vi "DOOR_ASSIGN.vi"(8 "error In":errorcluster) -> (0 "error out":errorcluster)   [LabVIEW 2017]
uses:
  Controls/Ass. Loop Control.ctl
  <vilib>/Utility/error.llb/DialogType.ctl
  <vilib>/Utility/file.llb/Read Delimited Spreadsheet (string).vi
  <vilib>/Utility/file.llb/Write Delimited Spreadsheet (string).vi
  <vilib>/Utility/config.llb/NI_LVConfig.lvlib
panel:
  in  "REMOVE PART":bool
  in  "ADD PART":bool
  in  "LIST OF PARTS":string(combo)
  in  "DOORS":string(combo)
  in  "DOORS":enum32{"ADD PARTS", "Page 1", "Page 2"}(tab)
  in  "ADDED PART LIST":string(combo)
  in  "REMOVE PART FROM LIST":bool
  in  "ADD PART IN LIST":bool
  in  "NEW PARTS BARCODE":string
  out "DOOR 1":string[](array[string])
  out "DOOR 2":string[](array[string])
  out "DOOR 3":string[](array[string])
  out "DOOR 4":string[](array[string])
  out "DOOR 5":string[](array[string])
  out "DOOR 16":string[](array[string])
  out "DOOR 11":string[](array[string])
  out "DOOR 12":string[](array[string])
  out "DOOR 13":string[](array[string])
  out "DOOR 14":string[](array[string])
  out "DOOR 15":string[](array[string])
  out "USER:-":string
  in  "Stop":bool
  out "DATE/TIME":string
  out "Screen Name":string
  # "Nm"
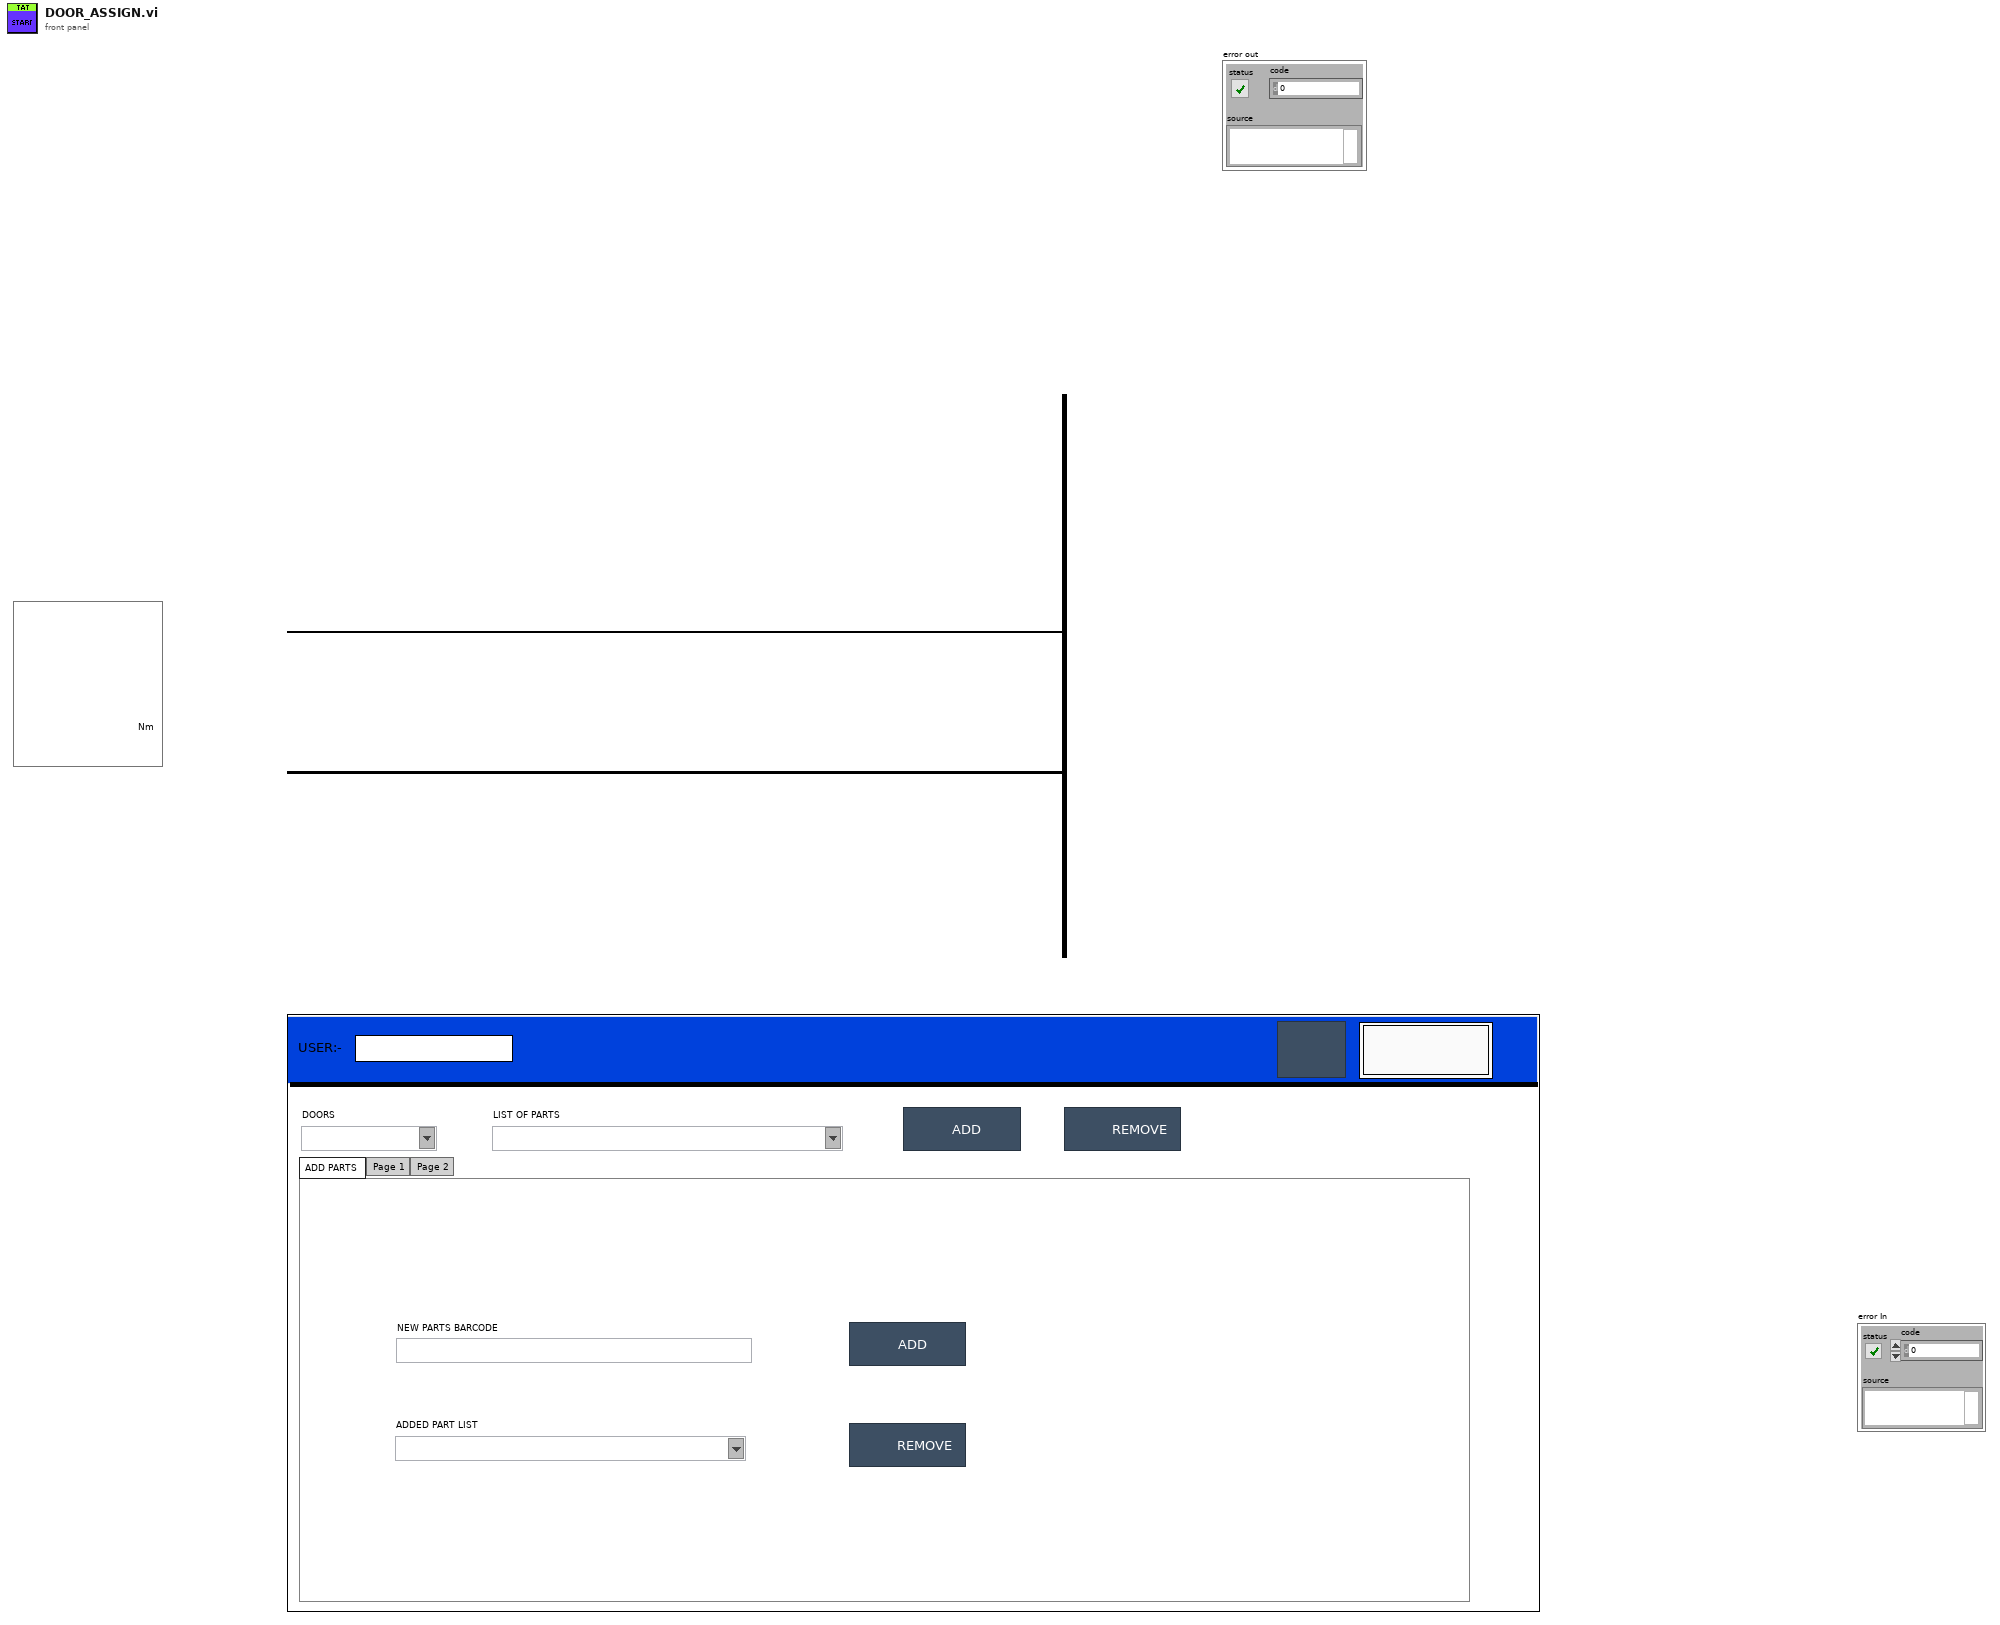
[diagram p1: front panel]
types:
  T1 = cluster{"DOOR ASSIGN":path, "PART LIST":path, "DOOR PART ASSIGN":cluster{"DOOR 1":cluster{"DOOR 1":string[]}, "DOOR 2":cluster{"DOOR 2":string[]}, "DOOR 3":cluster{"DOOR 3":string[]}, "DOOR 4":cluster{"DOOR 4":string[]}, "DOOR 5":cluster{"DOOR 5":string[]}, "DOOR 11":cluster{"DOOR 11":string[]}, "DOOR 12":cluster{"DOOR 12":string[]}, "DOOR 13":cluster{"DOOR 13":string[]}, "DOOR 14":cluster{"DOOR 14":string[]}, "DOOR 15":cluster{"DOOR 15":string[]}, "DOOR 16":cluster{"DOOR 16":string[]}}}
  T2 = typedef "Ass. Loop Control.ctl" = enum16{"Package_Qty_Count", "GENERATE_QR_PRNT", "Cluster_update", "Waiting_for_scan", "barcode CHECK", "Int", "SaveReport ", "Barcode Print", "Start Cycle", "Wait", "Cycle End", "Stop"}
  T3 = typedef "DialogType.ctl" = u16
  T4 = enum32{"invalid app kind", "Development System", "Run Time System", "Student Edition", "Embedded LabVIEW", "Evaluation", "Custom"}
  T5 = cluster{"DOOR 1":string[], "DOOR 2":string[], "DOOR 3":string[], "DOOR 4":string[], "DOOR 5":string[], "DOOR 11":string[], "DOOR 12":string[], "DOOR 13":string[], "DOOR 14":string[], "DOOR 15":string[], "DOOR 16":string[]}
  T6 = typedef "LVComboBoxStrsAndValuesArrayTypeDef.ctl" = cluster{"String":string, "Value":string}[]
  T7 = typedef "NI_LVConfig.lvlib/Config Data RefNum.ctl" = refnum<k1>
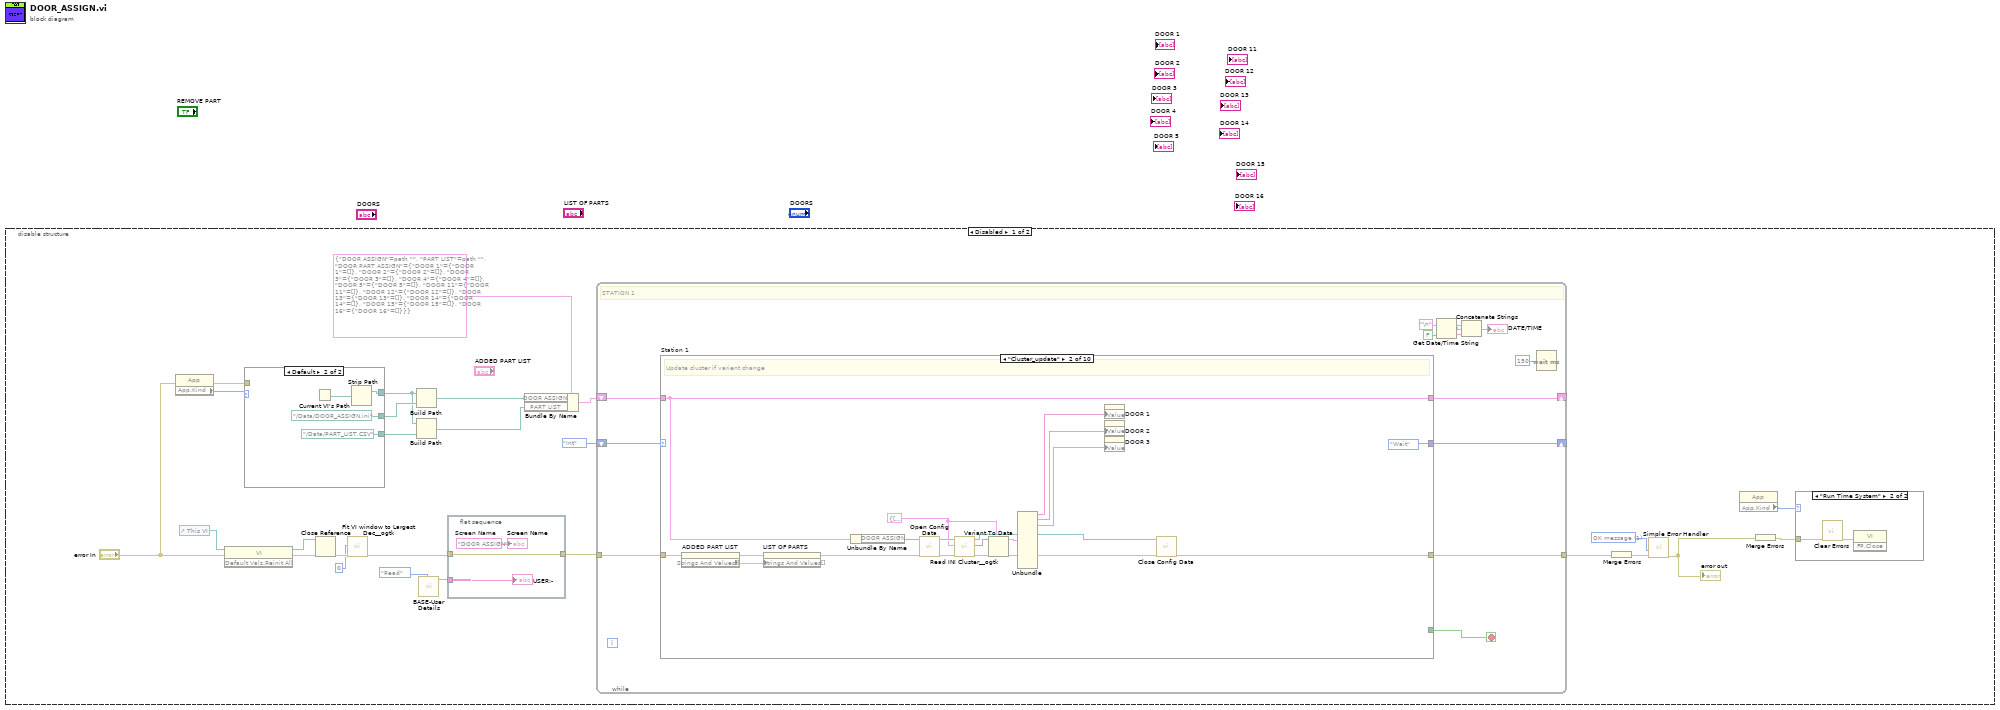
[diagram p0: block diagram]
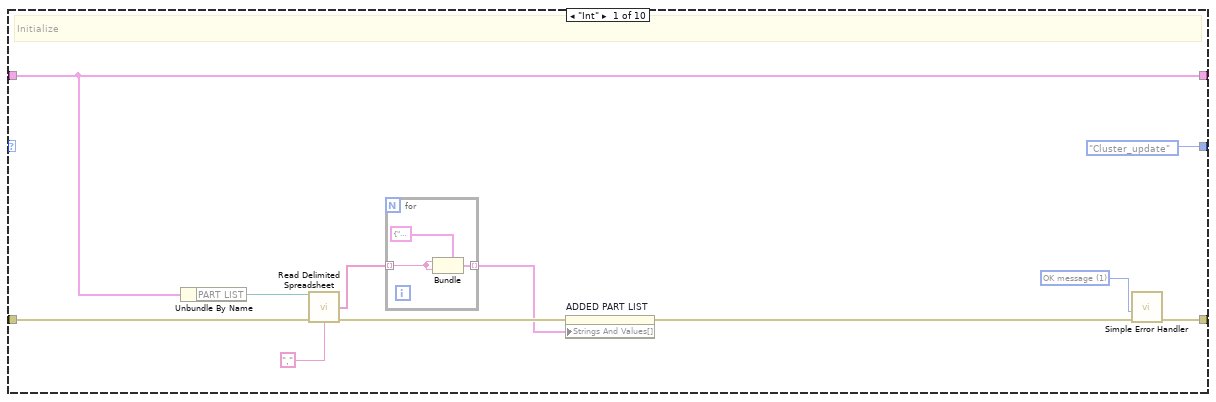
[diagram p3: hidden frame]
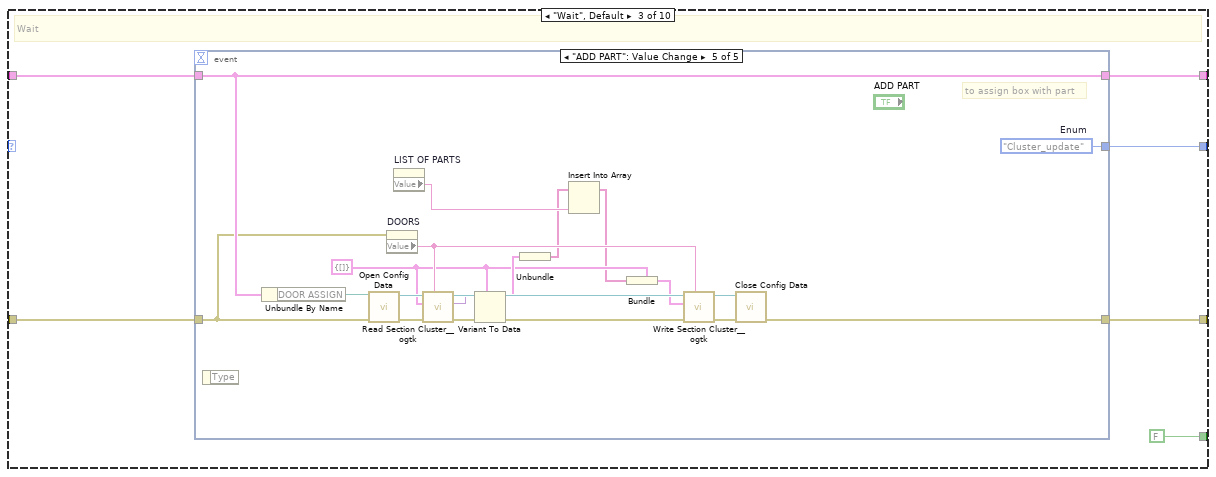
[diagram p4: hidden frame]
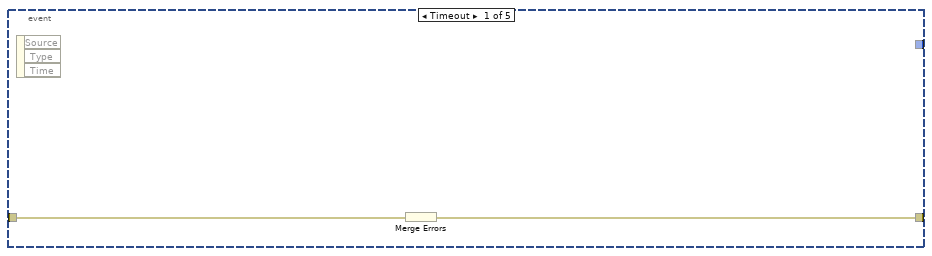
[diagram p5: hidden frame]
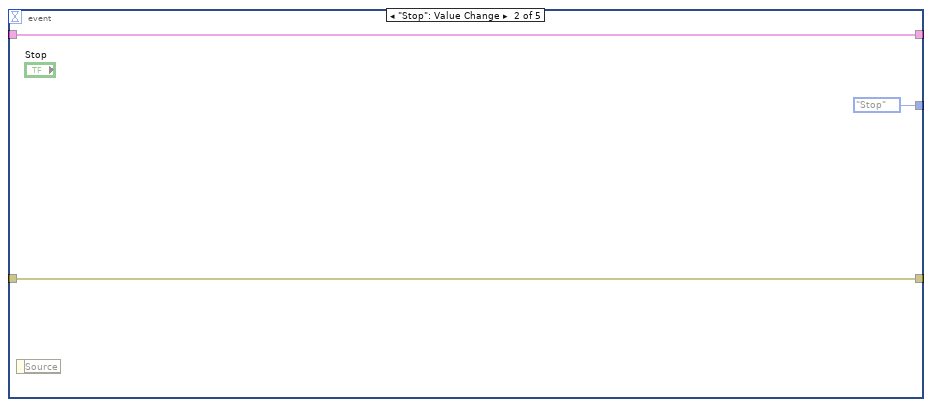
[diagram p6: hidden frame]
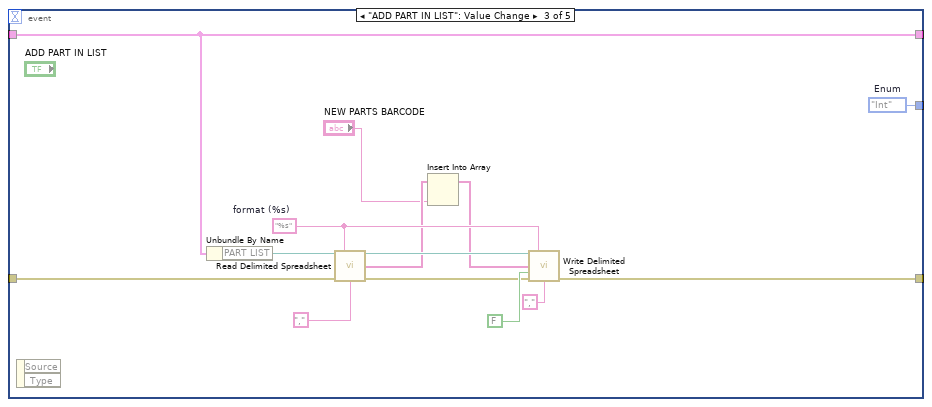
[diagram p7: hidden frame]
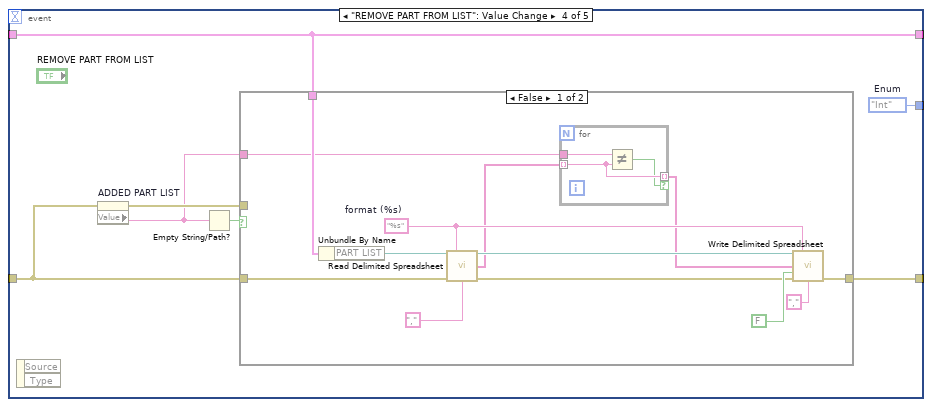
[diagram p8: hidden frame]
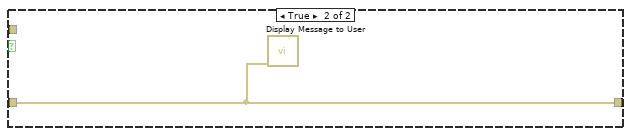
[diagram p9: hidden frame]
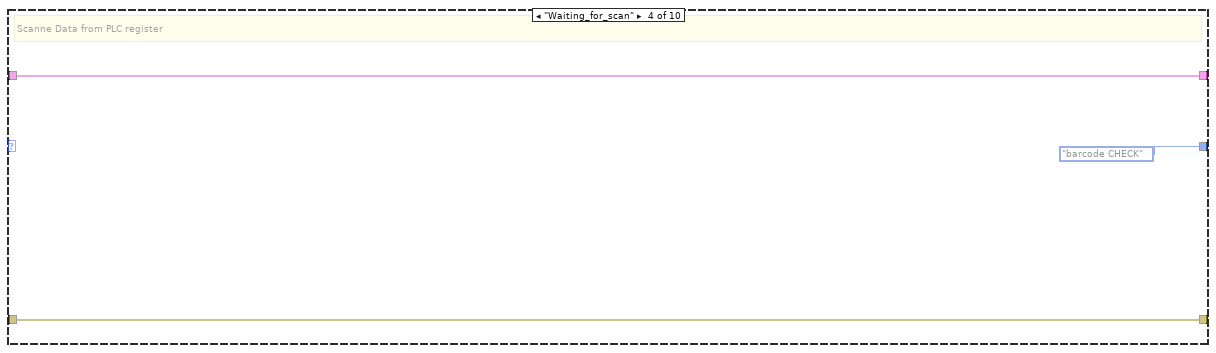
[diagram p10: hidden frame]
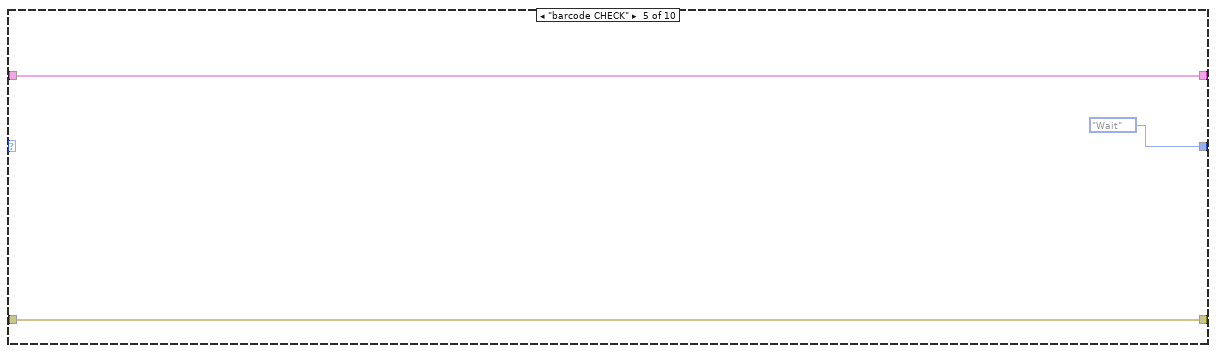
[diagram p11: hidden frame]
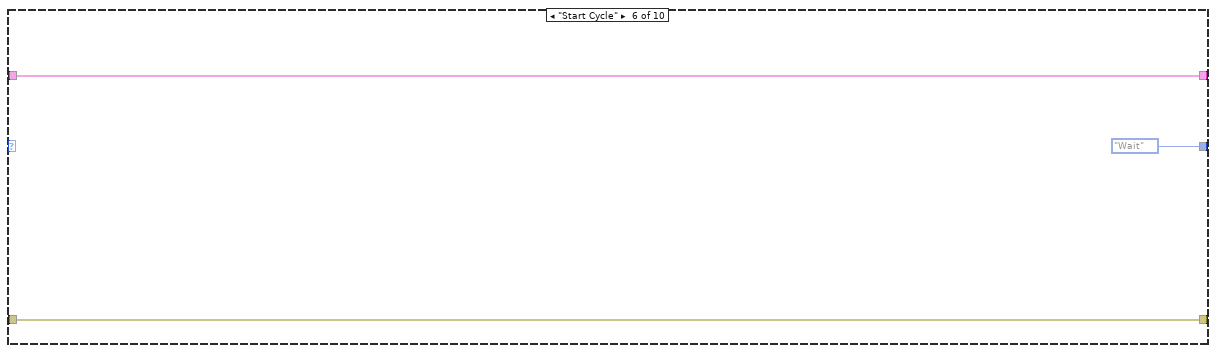
[diagram p12: hidden frame]
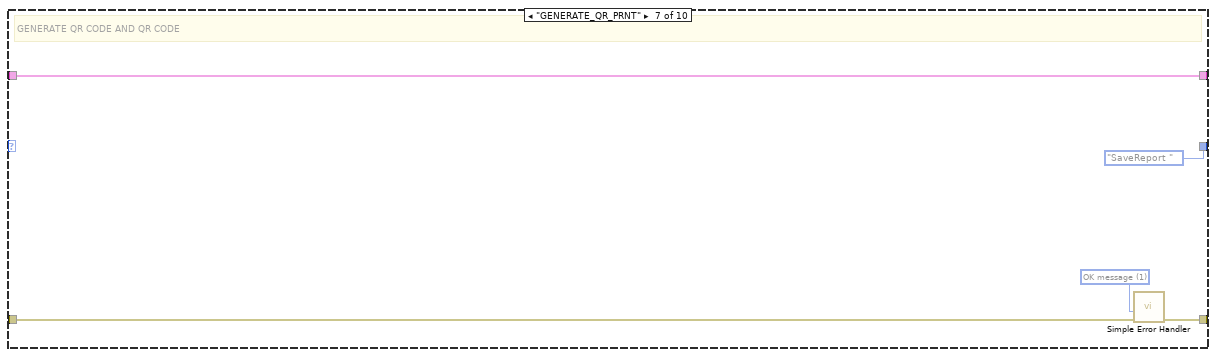
[diagram p13: hidden frame]
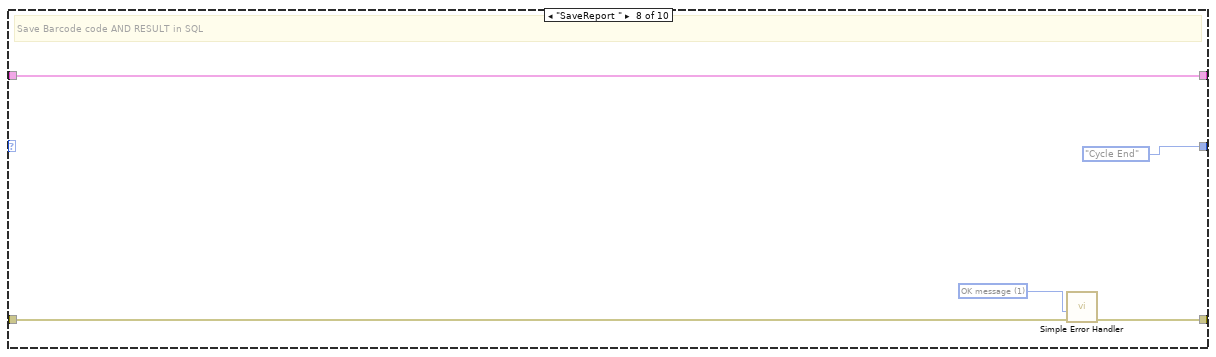
[diagram p14: hidden frame]
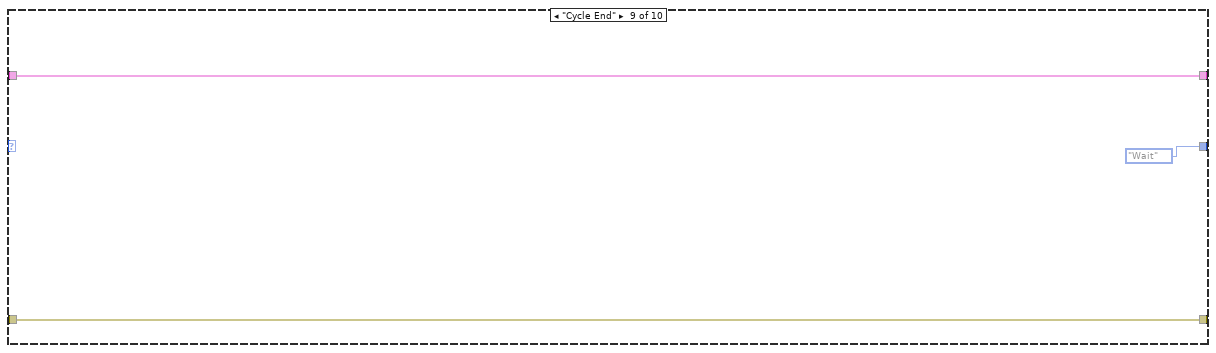
[diagram p15: hidden frame]
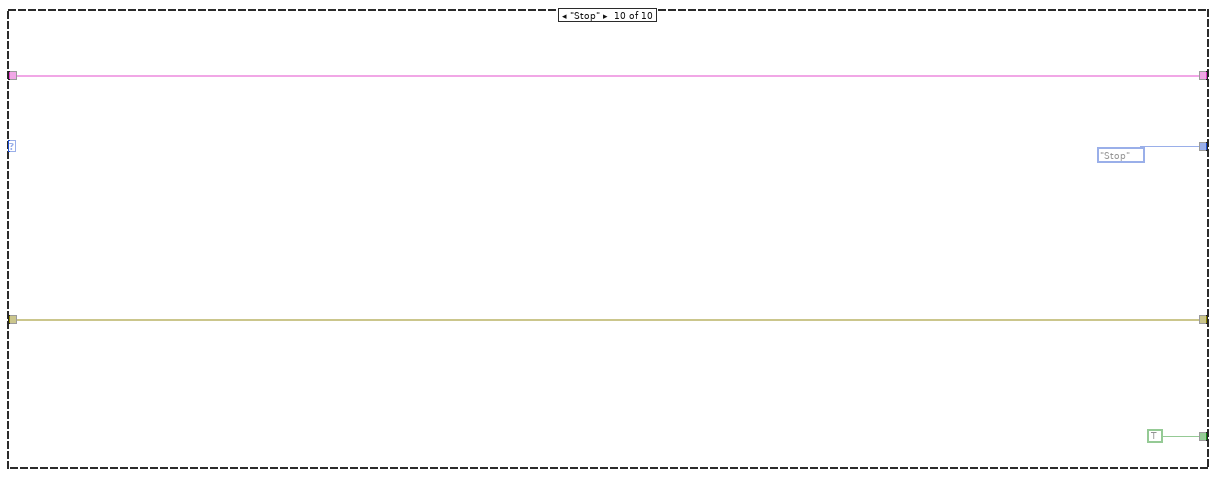
[diagram p16: hidden frame]
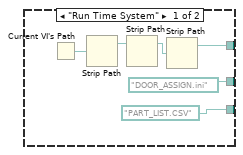
[diagram p17: hidden frame]
diagram:
  n1 = disable-structure shown="Disabled" {
    frame Disabled {
      w17 = T3 1 items=["no dialog", "OK message", "continue or stop message", "OK message + warnings", "continue/stop + warnings"] ("type of dialog (OK msg:1)")
      n2 = property class="App"(error in="error In") -> (error out=w13:errorcluster, "App.Kind"=w15:T4)  [unwired: 1 in, 1 out]
      n3 = control-ref of="This VI"() -> (w26:refnum<vi>)
      n4 = invoke class="VI" method="Default Vals.Reinit All"(reference=w26, error in="error In") -> (reference out=w24:refnum<vi>, error out=w25:errorcluster)  [unwired: 1 in, 1 out]
      n5 = case shown="Default" w15 {
        tunnel: [path "DOOR_ASSIGN.ini" ("path") path "../Data/DOOR_ASSIGN.ini" ("path")] -> w14
        tunnel: [w174 w180] -> w3
        tunnel: w13 -> [_ _]
        tunnel: [path "PART_LIST.CSV" ("path") path "../Data/PART_LIST.CSV" ("path")] -> w2
        frame "Run Time System" {
          n6 = Current VI's Path() -> (path=w177:path)
          n7 = Strip Path(path=w177) -> (stripped path=w176:path)  [unwired: 1 out]
          n8 = Strip Path(path=w176) -> (stripped path=w175:path)  [unwired: 1 out]
          n9 = Strip Path(path=w175) -> (stripped path=w174:path)  [unwired: 1 out]
        }
        frame Default {
          n10 = Current VI's Path() -> (path=w181:path)
          n11 = Strip Path(path=w181) -> (stripped path=w180:path)  [unwired: 1 out]
        }
      }
      n12 = Close Reference(reference=w24, error in (no error)=w25) -> (error out=w23:errorcluster)
      n13 = call <userlib>:"Fit VI window to Largest Dec__ogtk.vi"("error in (no error)"=w23, "border spacing (2 px)"=0) -> ("error out"=w11:errorcluster)  [unwired: 4 in, 1 out]
      n14 = Build Path(base path=w3, name or relative path=w14) -> (appended path=w4:path)
      n15 = Build Path(base path=w3, name or relative path=w2) -> (appended path=w1:path)
      n16 = call "BASE-User Details.vi"("Enum"=enum16{"Read", "Write"}."Read") -> ("User Name Out"=w18:string)  [unwired: 9 in, 1 out]
      n17 = flat-sequence {
        tunnel: [w29] -> w7
        tunnel: w11 -> [w29]
        tunnel: w18 -> [w28]
        frame #0 {
          w27 = "DOOR ASSIGN"  # Screen Name
          "USER:-" <- w28
          "Screen Name" <- w27
        }
      }
      n18 = Bundle By Name(cluster=T1 {"DOOR ASSIGN"=path "", "PART LIST"=path "", "DOOR PART ASSIGN"={"DOOR 1"={"DOOR 1"=[]}, "DOOR 2"={"DOOR 2"=[]}, "DOOR 3"={"DOOR 3"=[]}, "DOOR 4"={"DOOR 4"=[]}, "DOOR 5"={"DOOR 5"=[]}, "DOOR 11"={"DOOR 11"=[]}, "DOOR 12"={"DOOR 12"=[]}, "DOOR 13"={"DOOR 13"=[]}, "DOOR 14"={"DOOR 14"=[]}, "DOOR 15"={"DOOR 15"=[]}, "DOOR 16"={"DOOR 16"=[]}}}, "DOOR ASSIGN"=w4, "PART LIST"=w1) -> (w5:T1)
      n19 = while {
        tunnel: w7 -> [w34]
        shift-right: [w35] -> _
        shift-left: Ass._Loop_Control."Int" ("Enum") -> [w44]
        tunnel: [w42] -> w21
        shift-right: [w32] -> _
        shift-left: w5 -> [w33]
        stop <- w36 stop-if-true
        # "STATION 1"
        n20 = case "Station 1" shown="\"Cluster_update\"" w44 {
          tunnel: [Ass._Loop_Control."Cluster_update" ("Enum") Ass._Loop_Control."Wait" ("Enum") w80 Ass._Loop_Control."barcode CHECK" ("Enum") Ass._Loop_Control."Wait" ("Enum") Ass._Loop_Control."Wait" ("Enum") Ass._Loop_Control."SaveReport " ("Enum") Ass._Loop_Control."Cycle End" ("Enum") Ass._Loop_Control."Wait" ("Enum") Ass._Loop_Control."Stop" ("Enum")] -> w35
          tunnel: [_ _ FALSE _ _ _ _ _ _ TRUE] -> w36
          tunnel: [w53 w63 w81 w148 w151 w154 w159 w163 w167 w170] -> w42
          tunnel: w34 -> [w49 w74 w82 w148 w151 w154 w157 w162 w167 w170]
          tunnel: w33 -> [w51 w65 w78 w147 w150 w153 w156 w161 w166 w169]
          tunnel: [w51 w65 w79 w147 w150 w153 w156 w161 w166 w169] -> w32
          frame "Int" {
            w54 = T3 1 items=["no dialog", "OK message", "continue or stop message", "OK message + warnings", "continue/stop + warnings"] ("type of dialog (OK msg:1)")
            # "Initialize"
            n21 = Unbundle By Name(w51) -> ("PART LIST"=w50:path)
            n22 = call-poly <vilib>:"Read Delimited Spreadsheet.vi"("file path (dialog if empty)"=w50, "error in (no error)"=w49, "delimiter (\\t)"="," ("format (%s)")) -> ("first row"=w46:string[], "error out"=w48:errorcluster)  [unwired: 7 in, 4 out]
            n23 = for {
              tunnel: w46 -> [w57] mode=indexing
              tunnel: [w56] -> w45 mode=indexing
              n24 = Bundle(cluster=cluster{"String":string, "Value":string} {"String"="", "Value"=""}, "String"=w57, "Value"=w57) -> (w56:cluster{"String":string, "Value":string})
            }
            n25 = property on="ADDED PART LIST" class="CmbBox"(error in=w48, "Strings And Values[]"=w45) -> (error out=w52:errorcluster)  [unwired: 1 in, 1 out]
            n26 = call <vilib>:"Simple Error Handler.vi"("type of dialog (OK msg:1)"=w54, "error in (no error)"=w52) -> ("error out"=w53:errorcluster)  [unwired: 3 in, 4 out]
          }
          frame "Cluster_update" {
            w61 = T5 {"DOOR 1"=[], "DOOR 2"=[], "DOOR 3"=[], "DOOR 4"=[], "DOOR 5"=[], "DOOR 11"=[], "DOOR 12"=[], "DOOR 13"=[], "DOOR 14"=[], "DOOR 15"=[], "DOOR 16"=[]}
            # "Update cluster if varient change"
            n27 = property on="ADDED PART LIST" class="CmbBox"(error in=w74) -> (error out=w75:errorcluster, "Strings And Values[]"=w76:T6)  [unwired: 1 in, 1 out]
            n28 = property on="LIST OF PARTS" class="CmbBox"(error in=w75, "Strings And Values[]"=w76) -> (error out=w64:errorcluster)  [unwired: 1 in, 1 out]
            n29 = Unbundle By Name(w65) -> ("DOOR ASSIGN"=w73:path)
            n30 = call <vilib>:"Open Config Data.vi"("error in (no error)"=w64, "configuration file path"=w73) -> ("error out"=w72:errorcluster, "refnum"=w70:T7)  [unwired: 7 in, 1 out]
            n31 = call <userlib>:"Read INI Cluster__ogtk.vi"("error in (no error)"=w72, "INI Fomatted Cluster Type"=w61, "refnum"=w70) -> ("error out"=w68:errorcluster, "INI Fomatted Cluster"=w69:variant, "dup refnum"=w71:T7)  [unwired: 4 in, 2 out]
            n32 = Variant To Data(error in=w68, type=w61, Variant=w69) -> (data=w66:T5, error out=w67:errorcluster)
            n33 = Unbundle(w66) -> ("DOOR 1"=w62:string[], "DOOR 2"=w60:string[], "DOOR 3"=w59:string[])  [unwired: 8 out]
            n34 = property on="DOOR 1" class="Arr (strict)"("Value"=w62) -> ()  [unwired: 2 in, 2 out]
            n35 = property on="DOOR 2" class="Arr (strict)"("Value"=w60) -> ()  [unwired: 2 in, 2 out]
            n36 = property on="DOOR 3" class="Arr (strict)"("Value"=w59) -> ()  [unwired: 2 in, 2 out]
            n37 = call <vilib>:"Close Config Data.vi"("error in (no error)"=w67, "refnum"=w71) -> ("error out"=w63:errorcluster)  [unwired: 8 in, 1 out]
          }
          frame "Wait", Default {
            # "Wait"
            n38 = event shown="[4] \"ADD PART\": Value Change" {
              selector: _ -> [_ _ _ _ _]
              dyn-events: _ -> [_ _ _ _ _]
              timeout: _ -> [_ _ _ _ _]
              tunnel: w82 -> [w85 w87 w96 w106 w140]
              tunnel: [w84 w87 w95 w108 w144] -> w81
              tunnel: [_ Ass._Loop_Control."Stop" ("Enum") w89 w107 w143] -> w80
              tunnel: [_ w86 w100 w109 w142] -> w79
              tunnel: w78 -> [_ w86 w100 w109 w142]
              event Timeout {
                n39 = event-data() -> ()  [unwired: 1 in, 3 out]
                n40 = Merge Errors(w85) -> (w84:errorcluster)
              }
              event "Stop": Value Change {
                n41 = event-data() -> ()  [unwired: 1 in, 1 out]
              }
              event "ADD PART IN LIST": Value Change {
                w89 = Ass._Loop_Control."Int"  # Enum
                w93 = "%s"  # format (%s)
                n42 = event-data() -> ()  [unwired: 1 in, 2 out]
                n43 = Unbundle By Name(w100) -> ("PART LIST"=w102:path)
                n44 = call-poly <vilib>:"Read Delimited Spreadsheet.vi"("file path (dialog if empty)"=w102, "format (%s)"=w93, "error in (no error)"=w96, "delimiter (\\t)"="," ("format (%s)")) -> ("new file path (Not A Path if cancelled)"=w98:path, "first row"=w92:string[], "error out"=w97:errorcluster)  [unwired: 6 in, 3 out]
                n45 = Insert Into Array(array=w92, new element="NEW PARTS BARCODE") -> (w90:string[])  [unwired: 1 in]
                n46 = call-poly <vilib>:"Write Delimited Spreadsheet.vi"("file path (dialog if empty)"=w98, "format (%s)"=w93, "1D data"=w90, "append to file? (new file:F)"=FALSE, "error in (no error)"=w97, "delimiter (\\t)"="," ("format (%s)")) -> ("error out"=w95:errorcluster)  [unwired: 8 in, 1 out]
              }
              event "REMOVE PART FROM LIST": Value Change {
                w107 = Ass._Loop_Control."Int"  # Enum
                n47 = event-data() -> ()  [unwired: 1 in, 2 out]
                n48 = property on="ADDED PART LIST" class="CmbBox"(error in=w106) -> (error out=w104:errorcluster, "Value"=w103:string)  [unwired: 1 in, 1 out]
                n49 = Empty String/Path?(string/path=w103) -> (empty?=w105:bool)
                n50 = case shown="False" w105 {
                  tunnel: w109 -> [w120 _]
                  tunnel: [w116 w126] -> w108
                  tunnel: w106 -> [w113 w126]
                  tunnel: w104 -> [_ _]
                  tunnel: w103 -> [w111 _]
                  frame False {
                    w114 = "%s"  # format (%s)
                    n51 = Unbundle By Name(w120) -> ("PART LIST"=w122:path)
                    n52 = call-poly <vilib>:"Read Delimited Spreadsheet.vi"("file path (dialog if empty)"=w122, "format (%s)"=w114, "error in (no error)"=w113, "delimiter (\\t)"="," ("format (%s)")) -> ("new file path (Not A Path if cancelled)"=w118:path, "first row"=w112:string[], "error out"=w117:errorcluster)  [unwired: 6 in, 3 out]
                    n53 = for {
                      tunnel: w112 -> [w124] mode=indexing
                      tunnel: w111 -> [w125]
                      tunnel: [w124] -> w110 mode=indexing if=w123
                      n54 = Not Equal?(x=w125, y=w124) -> (x != y?=w123:bool)
                    }
                    n55 = call-poly <vilib>:"Write Delimited Spreadsheet.vi"("file path (dialog if empty)"=w118, "format (%s)"=w114, "1D data"=w110, "append to file? (new file:F)"=FALSE, "error in (no error)"=w117, "delimiter (\\t)"="," ("format (%s)")) -> ("error out"=w116:errorcluster)  [unwired: 8 in, 1 out]
                  }
                  frame True {
                    n56 = call "Display Message to User"("error in (no error)"=w126) -> ()  [unwired: 9 in, 2 out]
                  }
                }
              }
              event "ADD PART": Value Change {
                w129 = cluster{"BARCODE":string[]} {"BARCODE"=[]}
                w143 = Ass._Loop_Control."Cluster_update"  # Enum
                # "to assign box with part"
                n57 = event-data() -> ()  [unwired: 1 in, 1 out]
                n58 = Unbundle By Name(w142) -> ("DOOR ASSIGN"=w141:path)
                n59 = call <vilib>:"Open Config Data.vi"("error in (no error)"=w140, "configuration file path"=w141) -> ("error out"=w139:errorcluster, "refnum"=w137:T7)  [unwired: 7 in, 1 out]
                n60 = property on="DOORS" class="CmbBox"(error in=w140) -> ("Value"=w136:string)  [unwired: 1 in, 2 out]
                n61 = property on="LIST OF PARTS" class="CmbBox"() -> ("Value"=w132:string)  [unwired: 2 in, 2 out]
                n62 = call <userlib>:"Read Section Cluster__ogtk.vi"("section (optional)"=w136, "error in (no error)"=w139, "Section Formatted Cluster Type"=w129, "refnum"=w137) -> ("error out"=w134:errorcluster, "Section Formatted Cluster"=w135:variant, "dup refnum"=w138:T7)  [unwired: 3 in, 2 out]
                n63 = Variant To Data(error in=w134, type=w129, Variant=w135) -> (data=w131:cluster{"BARCODE":string[]}, error out=w133:errorcluster)
                n64 = Unbundle(w131) -> ("BARCODE"=w130:string[])
                n65 = Insert Into Array(array=w130, new element=w132) -> (w128:string[])  [unwired: 1 in]
                n66 = Bundle(cluster=w129, "BARCODE"=w128) -> (w127:cluster{"BARCODE":string[]})
                n67 = call <userlib>:"Write Section Cluster__ogtk.vi"("section (optional)"=w136, "error in (no error)"=w133, "Section Formatted Cluster"=w127, "refnum"=w138) -> ("error out"=w145:errorcluster, "dup refnum"=w146:T7)  [unwired: 6 in]
                n68 = call <vilib>:"Close Config Data.vi"("error in (no error)"=w145, "refnum"=w146) -> ("error out"=w144:errorcluster)  [unwired: 8 in, 1 out]
              }
            }
          }
          frame "Waiting_for_scan" {
            # "Scanne Data from PLC register"
          }
          frame "barcode CHECK" {
          }
          frame "Start Cycle" {
          }
          frame "GENERATE_QR_PRNT" {
            w160 = T3 1 items=["no dialog", "OK message", "continue or stop message", "OK message + warnings", "continue/stop + warnings"] ("type of dialog (OK msg:1)")
            # "GENERATE QR CODE AND QR CODE"
            n69 = call <vilib>:"Simple Error Handler.vi"("type of dialog (OK msg:1)"=w160, "error in (no error)"=w157) -> ("error out"=w159:errorcluster)  [unwired: 3 in, 4 out]
          }
          frame "SaveReport " {
            w164 = T3 1 items=["no dialog", "OK message", "continue or stop message", "OK message + warnings", "continue/stop + warnings"] ("type of dialog (OK msg:1)")
            # "Save Barcode code AND RESULT in SQL"
            n70 = call <vilib>:"Simple Error Handler.vi"("type of dialog (OK msg:1)"=w164, "error in (no error)"=w162) -> ("error out"=w163:errorcluster)  [unwired: 3 in, 4 out]
          }
          frame "Cycle End" {
          }
          frame "Stop" {
          }
        }
        n71 = Get Date/Time String(want seconds? (F)=FALSE) -> (date string=w40:string, time string=w39:string)  [unwired: 2 in]
        n72 = Concatenate Strings(w40, "\n", w39) -> (→"DATE/TIME":string)
        n73 = Wait (ms)(milliseconds to wait=u32 150) -> ()  [unwired: 1 out]
      }
      n74 = Merge Errors(w21) -> (w20:errorcluster)
      n75 = call <vilib>:"Simple Error Handler.vi"("type of dialog (OK msg:1)"=w17, "error in (no error)"=w20) -> ("error out"=w8:errorcluster)  [unwired: 3 in, 4 out]
      "error out" <- w8
      n76 = property class="App"() -> ("App.Kind"=w16:T4)  [unwired: 2 in, 2 out]
      n77 = Merge Errors(w8) -> (w9:errorcluster)
      n78 = case shown="\"Run Time System\"" w16 {
        tunnel: w9 -> [_ w31]
        frame "invalid app kind", Default {
        }
        frame "Run Time System" {
          n79 = call <vilib>:"Clear Errors.vi"("error in (no error)"=w31) -> ("error out"=w30:errorcluster)  [unwired: 5 in, 1 out]
          n80 = invoke class="VI" method="FP.Close"(error in=w30) -> ()  [unwired: 2 in, 3 out]
        }
      }
    }
    frame Enabled {
    }
  }
